vi "Target - Pass HTTP Get Data for Async Call.vi"(10 "Remote Port":u16=80, 11 "Address":string) -> (3 "Results":string)   [LabVIEW 2019]
doc: "This is a wrapper for the VI that sends an HTTP Get request. This VI can be used in conjunction with the Run VI method and will use a queue to return the results of the HTTP Get."
panel:
  # "This VI is used by Benchmarking Asynchronous Calls.vi."
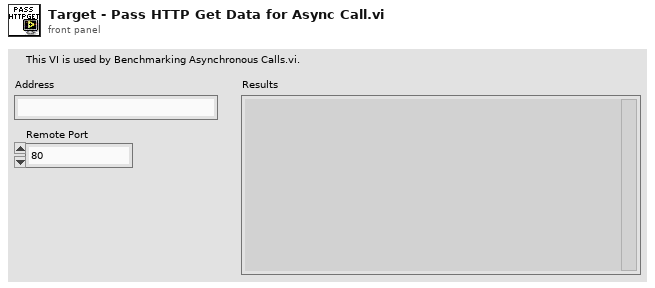
[diagram p1: front panel]
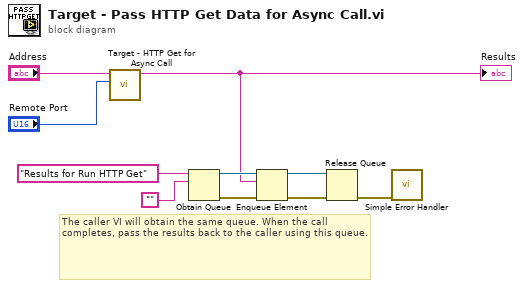
[diagram p0: block diagram]
diagram:
  # "The caller VI will obtain the same queue. When the call completes, pass the results back to the caller using this queue."
  n1 = call "Target - HTTP Get for Async Call.vi"("Remote Port"="Remote Port", "Address"="Address") -> ("Results"=w5:string)  [unwired: 9 in]
  "Results" <- w5
  n2 = Obtain Queue(name (unnamed)="Results for Run HTTP Get", element data type="") -> (queue out=w6:refnum<queue>, error out=w7:errorcluster)  [unwired: 3 in, 1 out]
  n3 = Enqueue Element(queue=w6, element=w5, error in (no error)=w7) -> (queue out=w3:refnum<queue>, error out=w2:errorcluster)  [unwired: 1 in, 1 out]
  n4 = Release Queue(queue=w3, error in (no error)=w2) -> (error out=w1:errorcluster)  [unwired: 1 in, 2 out]
  n5 = call <vilib>:"Simple Error Handler.vi"("error in (no error)"=w1) -> ()  [unwired: 4 in, 5 out]
